vi "Set IO Read State Ready Event.vi"(11 "dataevent":u32) -> (3 "dataevent out":u32)   [LabVIEW 2021, in "vmmso.lvlib"]
doc: "DLL_API void WINAPI SetIOReadStateReadyEvent(HANDLE dataevent);"
uses:
  vmmso.lvlib
  vmmso.dll
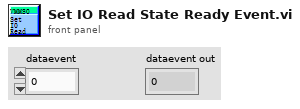
[diagram p1: front panel]
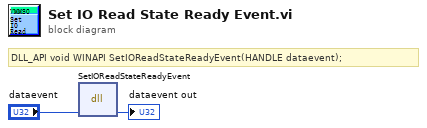
[diagram p0: block diagram]
diagram:
  # "DLL_API void WINAPI SetIOReadStateReadyEvent(HANDLE dataevent);"
  n1 = dll-call lib="D:/labviewdemo/LabviewDemo 21/vmmso/vmmso.*" fn="SetIOReadStateReadyEvent"("dataevent"="dataevent") -> ("dataevent"=→"dataevent out":u32)  [unwired: 4 in, 2 out]
